vi "I2CRxRead.vi"(8 "error in (no error)":errorcluster caption="错误输入（无错误）", 9 "addr":u8 format="%.0x", 10 "length":i32=256, 11 "handle":u64) -> (0 "error out":errorcluster caption="错误输出", 1 "rgRX":u8[](array[numeric]), 2 "function return":i32, 3 "handle out":u64, 4 "rxcount out":i32)   [LabVIEW 2018]
doc: "Set pos. or neg. Supply voltage"
panel:
  out "fParity out":i32
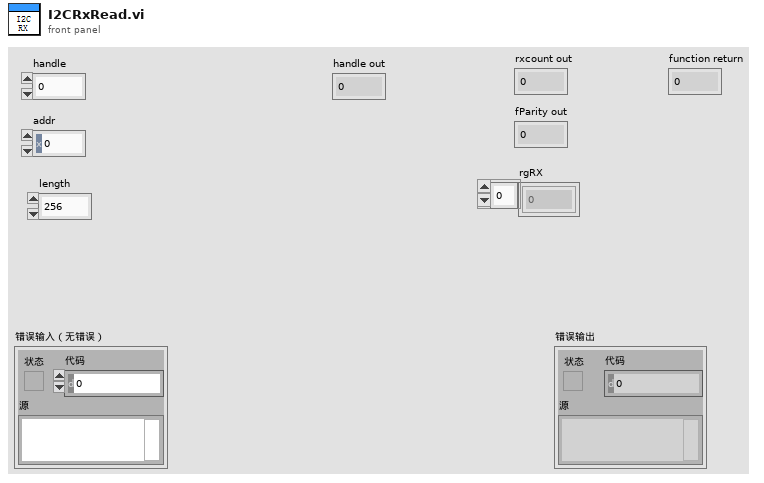
[diagram p1: front panel]
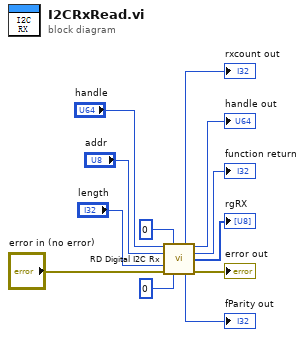
[diagram p0: block diagram]
diagram:
  n1 = call "RD Digital I2C Rx.vi"("handle"="handle", "rxcount"=0, "addr"="addr", "length"="length", "error in (no error)"="error in (no error)", "fParity"=0) -> ("rxcount out"=→"rxcount out":i32, "handle out"=→"handle out":u64, "function return"=→"function return":i32, "rgRX out"=→"rgRX":u8[], "fParity out"=→"fParity out":i32, "error out"=→"error out":errorcluster)  [unwired: 4 in]
